vi "Create User Event.vi"(8 "error in (no error)":errorcluster) -> (0 "error out":errorcluster, 3 "REQ Event":T1)   [LabVIEW 2021]
panel:
  in  "REQ Event":T1
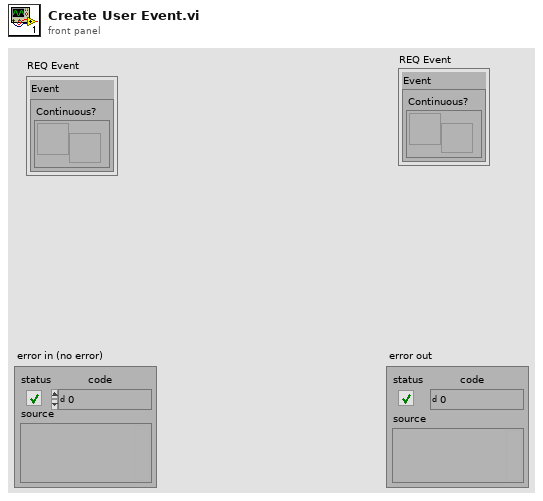
[diagram p1: front panel]
types:
  T1 = cluster{"Event":cluster{"Continuous?":refnum<user-event>}}
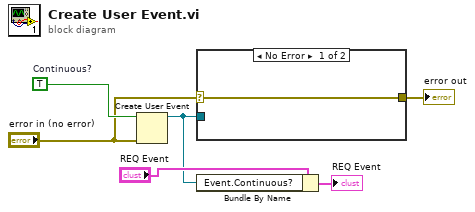
[diagram p0: block diagram]
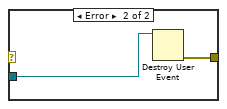
[diagram p2: hidden frame]
diagram:
  w6 = TRUE  # Continuous?
  n1 = Create User Event(user event datatype=w6, error in="error in (no error)") -> (user event=w3:refnum<user-event>)  [unwired: 1 out]
  n2 = case shown="No Error" "error in (no error)" {
    selector: "error in (no error)" -> [w7 _]
    tunnel: w3 -> [_ w9]
    tunnel: [w7 w8] -> w2
    frame No Error {
    }
    frame Error {
      n3 = Destroy User Event(user event=w9) -> (error out=w8:errorcluster)  [unwired: 1 in]
    }
  }
  "error out" <- w2
  n4 = Bundle By Name(cluster="REQ Event", "Event.Continuous?"=w3) -> (→"REQ Event":T1)
